vi "while_v0_v0.vi"() -> ()   [LabVIEW 2010]
panel:
  in  "stop":bool
  out "Numeric":dbl
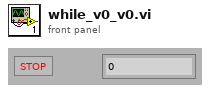
[diagram p1: front panel]
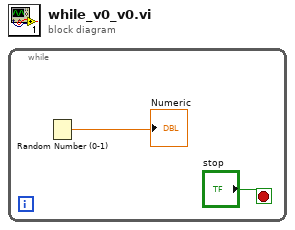
[diagram p0: block diagram]
diagram:
  n1 = while {
    stop <- "stop" stop-if-true
    n2 = Random Number (0-1)() -> (number: 0 to 1=→"Numeric":dbl)
  }
